vi "OE1022D_Configure Sensitivity.vi"(0 "VISA resource name":refnum<visa-resource-name>, 1 "OE1022D A/B":u8(ring) items=["Channel A", "Channel B"], 2 "Sensitivity":u16(ring)=24 items=["1 nV/fA", "2 nV/fA", "5 nV/fA", "10 nV/fA", "20 nV/fA", "50 nV/fA", "100 nV/fA", "200 nV/fA", "500 nV/fA", "1 uV/pA", "2 uV/pA", "5 uV/pA", "10 uV/pA", "20 uV/pA", "50 uV/pA", "100 uV/pA", "200 uV/pA", "500 uV/pA", "1 mV/nA", "2 mV/nA", "5 mV/nA", "10 mV/nA", "20 mV/nA", "50 mV/nA", "100 mV/nA", "200 mV/nA", "500 mV/nA", "1 V/uA"], 5 "error in (no error)":errorcluster) -> (14 "VISA resource name out":refnum<visa-resource-name>, 19 "error out":errorcluster)   [LabVIEW 2022 SP3]
doc: "Configures the reference source and the internal oscillator."
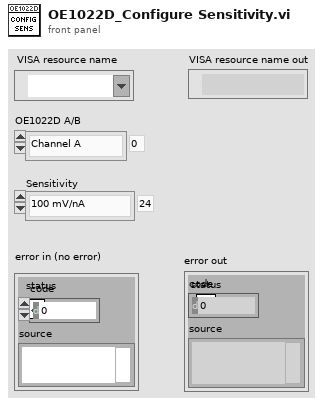
[diagram p1: front panel]
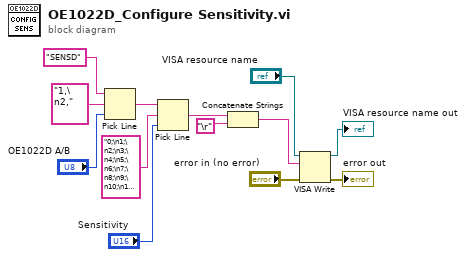
[diagram p0: block diagram]
diagram:
  n1 = Pick Line(string ("")="SENSD", multi-line string="1,\n2,", line index="OE1022D A/B") -> (output string=w13:string)
  n2 = Pick Line(string ("")=w13, multi-line string="0;\n1;\n2;\n3;\n4;\n5;\n6;\n7;\n8;\n9;\n10;\n11;\n12;\n13;\n14;\n15;\n16;\n17;\n18;\n19;\n20;\n21;\n22;\n23;\n24;\n25;\n26;\n27;", line index="Sensitivity") -> (output string=w2:string)
  n3 = Concatenate Strings(w2, "\r") -> (w1:string)
  n4 = VISA Write(VISA resource name="VISA resource name", write buffer=w1, error in (no error)="error in (no error)") -> (VISA resource name out=→"VISA resource name out":refnum<visa-resource-name>, error out=→"error out":errorcluster)  [unwired: 1 out]
